vi "Highlight Row.vi"(8 "Error In":errorcluster, 9 "Cell BG Color":u32(colorbox)=16759552, 10 "Row":i32, 11 "Table Ref":refnum<vi>) -> (0 "Error Out":errorcluster)   [LabVIEW 2019, in "Table Tools.lvlib"]
doc: "Highlight row in Table."
uses:
  Table Tools.lvlib
  <vilib>/Utility/miscctls.llb/LVRowAndColumnTypeDef.ctl
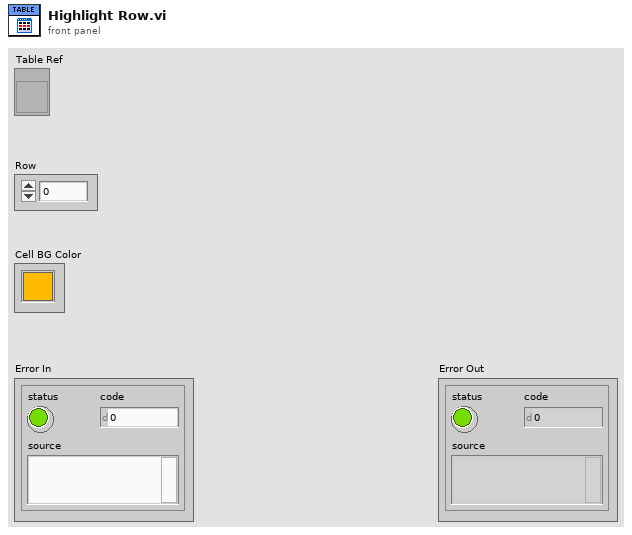
[diagram p1: front panel]
types:
  T1 = typedef "LVRowAndColumnTypeDef.ctl" = cluster{"Row":i32, "Column":i32}
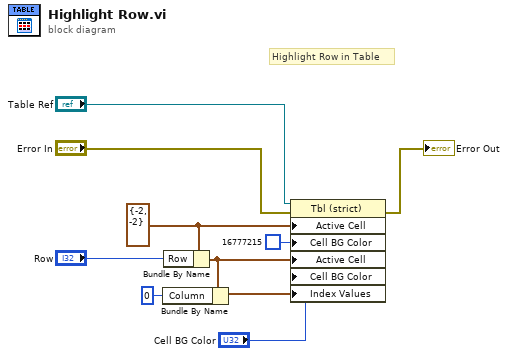
[diagram p0: block diagram]
diagram:
  w9 = T1 {"Row"=-2, "Column"=-2} ("Active Cell:Active Cell")
  # "Highlight Row in Table"
  n1 = Bundle By Name(cluster=w9, "Row"="Row") -> (w7:T1)
  n2 = Bundle By Name(cluster=w7, "Column"=0) -> (w6:T1)
  n3 = property class="Tbl (strict)"(reference="Table Ref", error in="Error In", "Active Cell"=w9, "Cell BG Color"=u32 16777215, "Active Cell"=w7, "Cell BG Color"="Cell BG Color", "Index Values"=w6) -> (error out=→"Error Out":errorcluster)  [unwired: 1 out]
